vi "Digital Write.vi"(8 "Error In":errorcluster, 10 "Digital Values":T1[](array[typedef]), 11 "LINX Device Config":T2) -> (0 "Error Out":errorcluster, 3 "LINX Device Config":T2)   [LabVIEW 2011, in "LVH-LINX.lvlib"]
doc: "Set the value of one or more digital output pin."
uses:
  LVH-LINX.lvlib
  Type Defs/LINX Device Config.ctl
  Type Defs/Interface.ctl
  Type Defs/TCP Config.ctl
  Type Defs/Peripherals/Digital/Digital Write Control.ctl
  Type Defs/Error Type.ctl
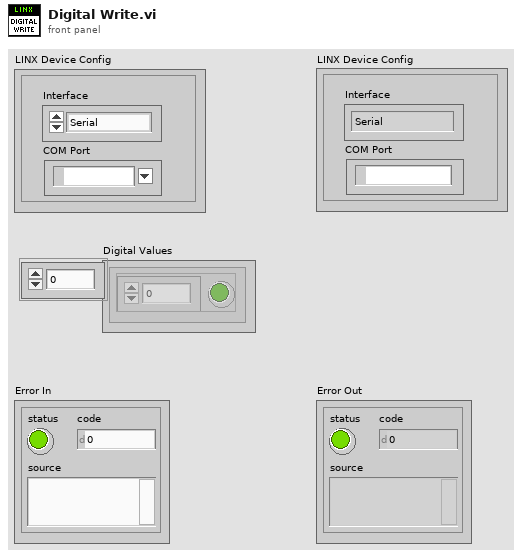
[diagram p1: front panel]
types:
  T1 = typedef "LVH-LINX.lvlib/Digital Write Control.ctl" = cluster{"Pin Number":u8, "Value":bool}
  T2 = typedef "LVH-LINX.lvlib/LINX Device Config.ctl" = cluster{"Interface":T3, "COM Port":refnum<visa-resource-name>, "Packet Number":u16, "TCP Configuration":T4}
  T3 = typedef "LVH-LINX.lvlib/Interface.ctl" = enum16{"Serial", "TCP"}
  T4 = typedef "LVH-LINX.lvlib/TCP Config.ctl" = cluster{"IP Address":string, "Port":dbl}
  T5 = typedef "LVH-LINX.lvlib/Error Type.ctl" = enum16{"Unknown", "Timeout", "Corrupt Return Packet", "Unable To Connect", "Command Not Supported"}
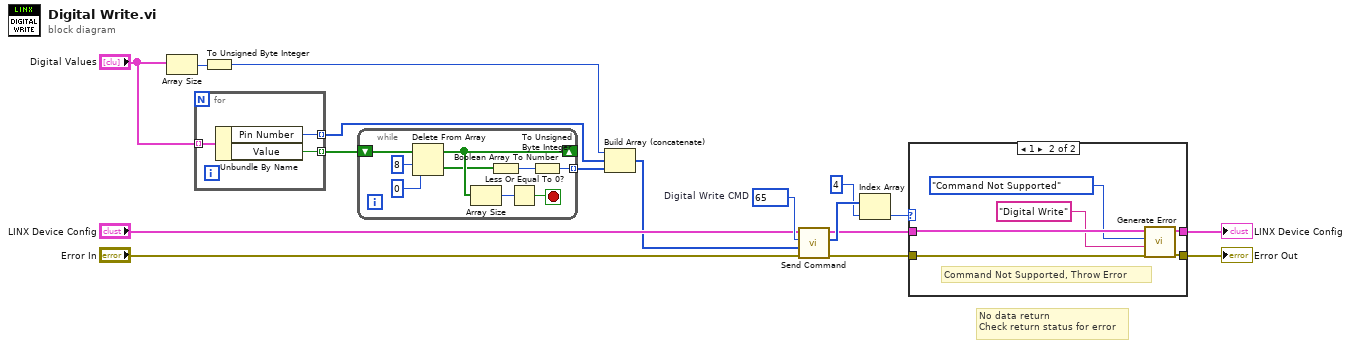
[diagram p0: block diagram]
diagram:
  w16 = u16 65  # Digital Write CMD
  # "No data return\nCheck return status for error"
  n1 = Array Size(array="Digital Values") -> (size(s)=w11:i32)
  n2 = for {
    tunnel: "Digital Values" -> [w20] mode=indexing
    tunnel: [w19] -> w12 mode=indexing
    tunnel: [w18] -> w13 mode=indexing
    n3 = Unbundle By Name(w20) -> ("Pin Number"=w19:u8, "Value"=w18:bool)
  }
  n4 = To Unsigned Byte Integer(number=w11) -> (unsigned 8bit integer=w10:u8)
  n5 = while {
    shift-right: [w26] -> _
    shift-left: w13 -> [w29]
    tunnel: [w21] -> w8 mode=indexing
    stop <- w24 stop-if-true
    n6 = Delete From Array(array=w29, length=8 ("index"), index=0 ("length")) -> (deleted portion=w23:bool[], array with subset deleted=w26:bool[])
    n7 = Array Size(array=w26) -> (size(s)=w25:i32)
    n8 = Boolean Array To Number(Boolean array=w23) -> (number=w22:u32)
    n9 = Less Or Equal To 0?(x=w25) -> (x <= 0?=w24:bool)
    n10 = To Unsigned Byte Integer(number=w22) -> (unsigned 8bit integer=w21:u8)
  }
  n11 = Build Array (concatenate)(w10, w12, w8) -> (w9:u8[])
  n12 = call "Send Command.vi"("Error In"="Error In", "ARGS"=w9, "CMD"=w16, "LINX Device Config"="LINX Device Config") -> ("Error Out"=w1:errorcluster, "Packet"=w7:u8[], "LINX Device Config"=w3:T2)  [unwired: 5 in]
  n13 = Index Array(array=w7, index=4) -> (element=w5:u8)
  n14 = case shown="1" w5 {
    tunnel: [w31 w34] -> w4
    tunnel: w3 -> [w31 w37]
    tunnel: [w30 w35] -> w2
    tunnel: w1 -> [w30 w36]
    frame 0, Default {
      # "Status OK"
    }
    frame 1 {
      # "Command Not Supported, Throw Error"
      n15 = call "Generate Error.vi"("Error In"=w36, "Arguments"="Digital Write", "Error Type"=Error_Type."Command Not Supported", "LINX Device Config"=w37) -> ("Error Out"=w35:errorcluster, "LINX Device Config"=w34:T2)  [unwired: 6 in]
    }
  }
  "Error Out" <- w2
  "LINX Device Config" <- w4
